vi "setBankingTransactionCategory.vi"(8 "error in (no error)":errorcluster, 9 "Transaction Ref":string, 10 "Category.lvclass":refnum<class "Category.lvclass">, 11 "Database in":refnum<class "Account History.lvclass">) -> (0 "error out":errorcluster, 3 "Database out":refnum<class "Account History.lvclass">)   [LabVIEW 2018, in "Account History.lvclass"]
uses:
  Account History.lvclass
  Category/Category.lvclass
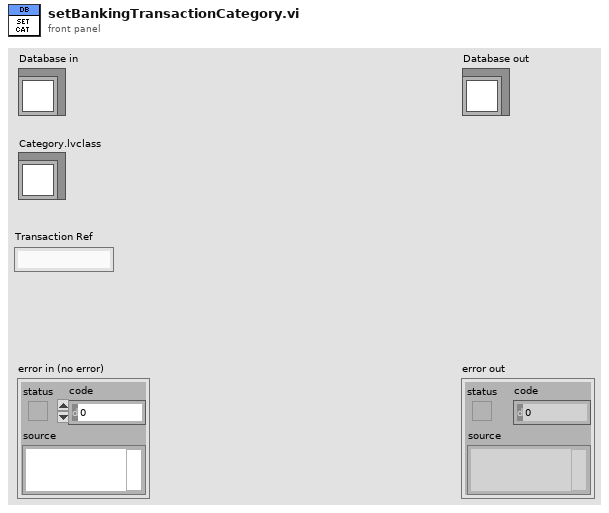
[diagram p1: front panel]
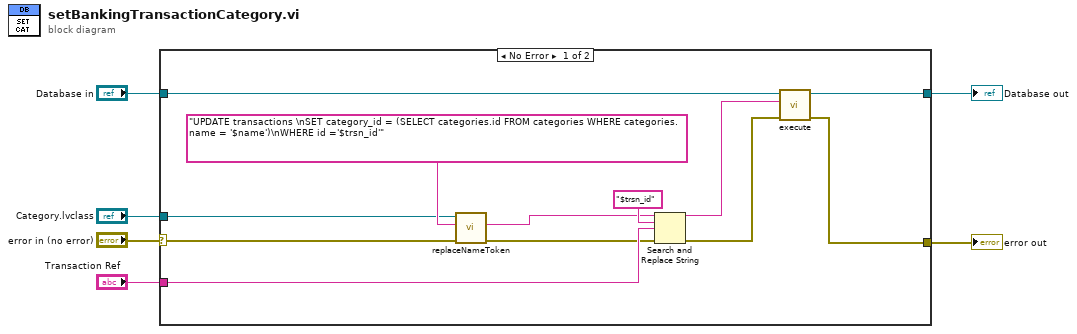
[diagram p0: block diagram]
diagram:
  n1 = case shown="No Error" "error in (no error)" {
    selector: "error in (no error)" -> [w7 w20]
    tunnel: [w16 w20] -> w5
    tunnel: [w18 w19] -> w3
    tunnel: "Database in" -> [w17 w19]
    tunnel: "Transaction Ref" -> [w12 _]
    tunnel: "Category.lvclass" -> [w8 _]
    frame No Error {
      n2 = call "replaceNameToken.vi"("error in (no error)"=w7, "Query In"="UPDATE transactions \nSET category_id = (SELECT categories.id FROM categories WHERE categories.name = '$name')\nWHERE id ='$trsn_id'", "Category in"=w8) -> ("error out"=w11:errorcluster, "Query Out"=w9:string)  [unwired: 6 in, 1 out]
      n3 = Search and Replace String(input string=w9, search string="$trsn_id", replace string=w12, error in=w11) -> (result string=w14:string, error out=w13:errorcluster)  [unwired: 4 in, 2 out]
      n4 = call "execute.vi"("error in (no error)"=w13, "SQL query"=w14, "Database in"=w17) -> ("error out"=w16:errorcluster, "Database out"=w18:refnum<class "Account History.lvclass">)  [unwired: 7 in]
    }
    frame Error {
    }
  }
  "error out" <- w5
  "Database out" <- w3
